vi "ZE_Recorder_ChoseToKeepTempConfig.vi"(8 "error in":errorcluster, 11 "channel config array":T1[](array[typedef])) -> (0 "error out":errorcluster, 3 "Keep Config?":bool=TRUE)   [LabVIEW 2025, in "ZE_Recorder.lvlib"]
doc: "ZE_Recorder_ChoseTempChannelType.vi\n----------------------------------------------\n\n\nInputs:\n---------------------\n- error in : Cluster; \n- channel name : String; \n\nOutputs:\n---------------------\n- error out : Cluster; \n- Cluster : Cluster; \n\n----------------------------------------------\n22.05.2017\nZühlke Engineering AG\nCH-8952 Schlieren\nwww.zuehlke.com"
uses:
  ZE_Recorder.lvlib
  ZE_Recorder_TempConfigCluster.ctl
  ZE_Recorder_TempParam.ctl
  ZE_Recorder_TempType.ctl
panel:
  in  "New Config":bool caption="Config OK"
  out "Info":string
  in  "Keep Config":bool caption="Config OK"
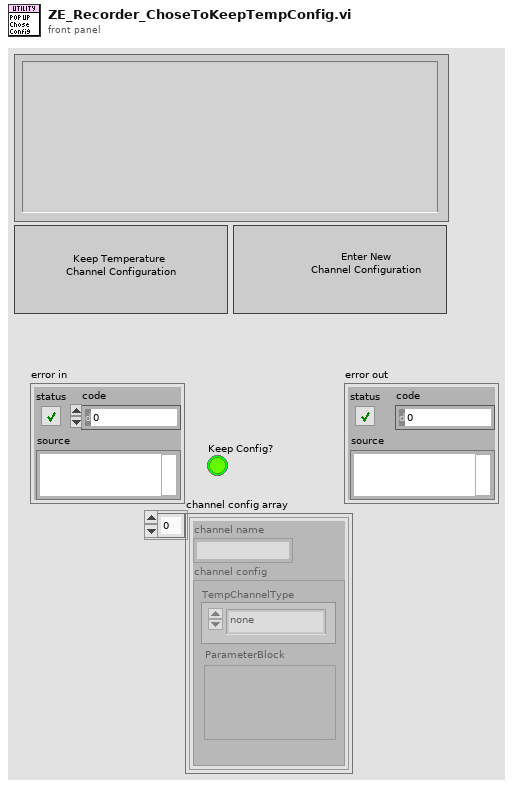
[diagram p1: front panel]
types:
  T1 = typedef "ZE_Recorder.lvlib/ZE_Recorder_TempConfigCluster.ctl" = cluster{"channel name":string, "channel config":T2}
  T2 = typedef "ZE_Recorder.lvlib/ZE_Recorder_TempParam.ctl" = cluster{"ParameterBlock":variant, "TempChannelType":T3}
  T3 = typedef "ZE_Recorder.lvlib/ZE_Recorder_TempType.ctl" = enum16{"none", "Thermocouple", "RTD", "Thermistor VE", "Thermistor CE"}
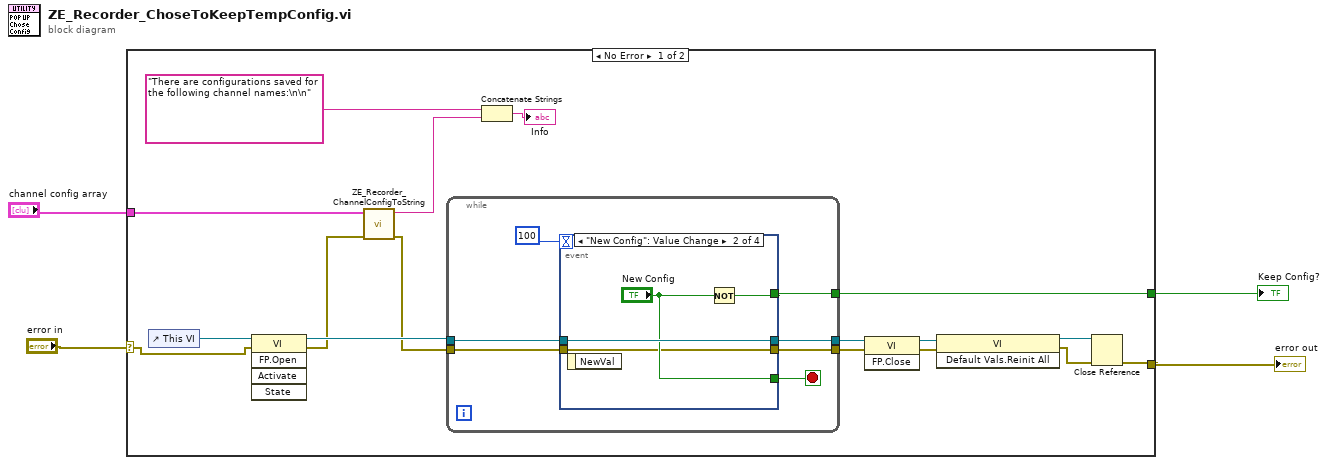
[diagram p0: block diagram]
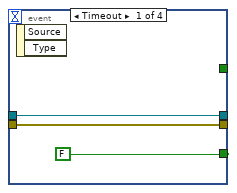
[diagram p2: hidden frame]
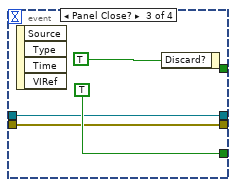
[diagram p3: hidden frame]
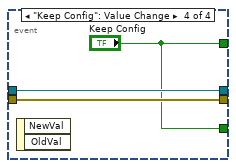
[diagram p4: hidden frame]
diagram:
  n1 = case shown="No Error" "error in" {
    selector: "error in" -> [w12 w43]
    tunnel: [w17 w43] -> w3
    tunnel: "channel config array" -> [w10 _]
    tunnel: [w7 _] -> w2
    frame No Error {
      n2 = control-ref of="This VI"() -> (w20:refnum<vi>)
      n3 = invoke class="VI" method="FP.Open"(reference=w20, error in=w12) -> (reference out=w19:refnum<vi>, error out=w6:errorcluster)  [unwired: 3 in, 3 out]
      n4 = call "ZE_Recorder_ChannelConfigToString.vi"("error in"=w6, "channel config array"=w10) -> ("error out"=w5:errorcluster, "Config String"=w9:string)  [unwired: 8 in]
      n5 = while {
        tunnel: w19 -> [w27]
        tunnel: w5 -> [w28]
        tunnel: [w25] -> w16
        tunnel: [w24] -> w18
        tunnel: [w22] -> w7
        stop <- w26 stop-if-true
        n6 = event shown="[1] \"New Config\": Value Change" {
          selector: _ -> [_ _ _ _]
          dyn-events: _ -> [_ _ _ _]
          timeout: 100 -> [_ _ _ _]
          tunnel: w28 -> [w31 w32 w38 w41]
          tunnel: w27 -> [w30 w35 w37 w42]
          tunnel: [w30 w35 w37 w42] -> w24
          tunnel: [FALSE "New Config" TRUE "Keep Config"] -> w26
          tunnel: [w31 w32 w38 w41] -> w25
          tunnel: [_ w34 _ "Keep Config"] -> w22
          event Timeout {
            n7 = event-data() -> ()  [unwired: 1 in, 2 out]
          }
          event "New Config": Value Change {
            n8 = event-data() -> ()  [unwired: 1 in, 1 out]
            n9 = Not(x="New Config") -> (.not. x?=w34:bool)
          }
          event Panel Close? {
            n10 = event-data() -> ()  [unwired: 1 in, 4 out]
            n11 = event-data("Discard?"=TRUE) -> ()  [unwired: 1 in, 1 out]
          }
          event "Keep Config": Value Change {
            n12 = event-data() -> ()  [unwired: 1 in, 2 out]
          }
        }
      }
      n13 = Concatenate Strings("There are configurations saved for the following channel names:\n\n", w9) -> (→"Info":string)
      n14 = invoke class="VI" method="FP.Close"(reference=w18, error in=w16) -> (reference out=w15:refnum<vi>, error out=w13:errorcluster)  [unwired: 1 in, 1 out]
      n15 = invoke class="VI" method="Default Vals.Reinit All"(reference=w15, error in=w13) -> (reference out=w14:refnum<vi>, error out=w11:errorcluster)  [unwired: 1 in, 1 out]
      n16 = Close Reference(reference=w14, error in (no error)=w11) -> (error out=w17:errorcluster)
    }
    frame Error {
    }
  }
  "error out" <- w3
  "Keep Config?" <- w2
